vi "Choose Axis.vi"(0 "sp in":dbl, 11 "Axis":enum16{"large axis", "small axis"}(ring)) -> (4 "axis 1: sp":dbl, 6 "move axis 1":bool, 8 "axis 2: sp":dbl, 10 "move axis 2":bool)   [LabVIEW 2016]
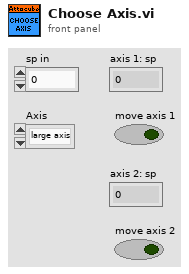
[diagram p1: front panel]
types:
  T1 = cluster{"axis 1: Current position (°)":dbl, "axis 2: Current position (°)":dbl, "axis 1: rot. count":dbl, "axis 2: rot. count":dbl, "axis 1: StepWidth":dbl, "axis 2: StepWidth":dbl, "axis 1: speed (°/s)":dbl, "axis 2: speed (°/s)":dbl, "axis 1: positioner status":cluster{"moving":bool, "stop detected":bool, "sensor error":bool, "sensor disconnected":bool}, "axis 2: positioner status":cluster{"moving":bool, "stop detected":bool, "sensor error":bool, "sensor disconnected":bool}}
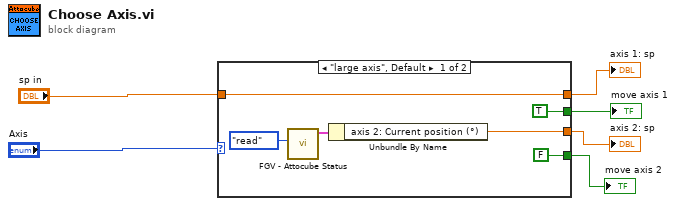
[diagram p0: block diagram]
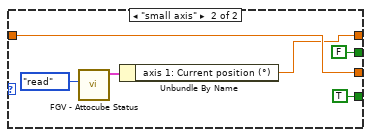
[diagram p2: hidden frame]
diagram:
  n1 = case shown="\"large axis\", Default" "Axis" {
    tunnel: [w10 w14] -> w1
    tunnel: [FALSE ("move axis 2") TRUE ("move axis 2")] -> w6
    tunnel: [TRUE ("move axis 1") FALSE ("move axis 1")] -> w5
    tunnel: [w7 w13] -> w4
    tunnel: "sp in" -> [w7 w14]
    frame "large axis", Default {
      n2 = call "FGV - Attocube Status.vi"("Function"=enum16{"write", "read"}."read") -> ("Status OUT"=w11:T1)  [unwired: 5 in, 1 out]
      n3 = Unbundle By Name(w11) -> ("axis 2: Current position (°)"=w10:dbl)
    }
    frame "small axis" {
      n4 = call "FGV - Attocube Status.vi"("Function"=enum16{"write", "read"}."read") -> ("Status OUT"=w17:T1)  [unwired: 5 in, 1 out]
      n5 = Unbundle By Name(w17) -> ("axis 1: Current position (°)"=w13:dbl)
    }
  }
  "move axis 2" <- w6
  "axis 2: sp" <- w1
  "move axis 1" <- w5
  "axis 1: sp" <- w4
